vi "Nudge__LCR.vi"(7 "Nudging?":bool, 8 "error in (no error)":errorcluster, 9 "Nudge?":bool, 10 "NudgeValue":i32=1, 11 "Pict In":refnum<vi>) -> (0 "error out":errorcluster, 3 "PictOut":refnum<vi>)   [LabVIEW 2011, in "BooleanXControl__LCR.xctl"]
doc: "This VI will move the picture when needed to suggest a nudge."
uses:
  BooleanXControl__LCR.xctl
  <vilib>/Utility/miscctls.llb/LVPointTypeDef.ctl
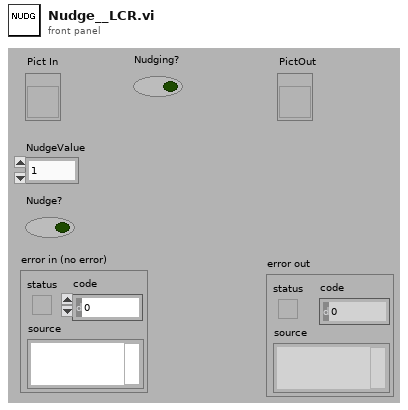
[diagram p1: front panel]
types:
  T1 = typedef "LVPointTypeDef.ctl" = cluster{"Horizontal":i16, "Vertical":i16}
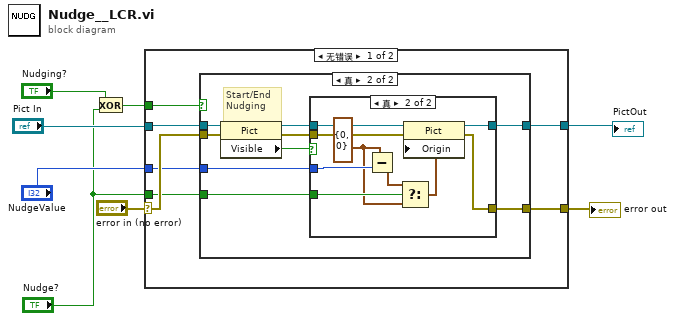
[diagram p0: block diagram]
diagram:
  n1 = Exclusive Or(1:"Nudge?", 2:"Nudging?") -> (0:w1:bool)
  n2 = case shown="无错误" "error in (no error)" {
    selector: "error in (no error)" -> [w14 w39]
    tunnel: [w12 w39] -> w7
    tunnel: "Pict In" -> [w15 w38]
    tunnel: "NudgeValue" -> [w13 _]
    tunnel: "Nudge?" -> [w11 _]
    tunnel: [w10 w38] -> w4
    tunnel: w1 -> [w9 _]
    frame No Error {
      n3 = case shown="真" w9 {
        tunnel: w15 -> [w17 w26]
        tunnel: w14 -> [w16 w25]
        tunnel: w13 -> [_ w21]
        tunnel: [w16 w20] -> w12
        tunnel: w11 -> [_ w19]
        tunnel: [w17 w18] -> w10
        frame False {
          # "Nudging status didn't change"
        }
        frame True {
          # "Start/End\nNudging"
          n4 = property class="Pict"(reference=w26, error in=w25) -> (reference out=w23:refnum<vi>, error out=w22:errorcluster, "Visible"=w24:bool)
          n5 = case shown="真" w24 {
            tunnel: w23 -> [w27 w35]
            tunnel: w22 -> [w28 w34]
            tunnel: w21 -> [_ w37]
            tunnel: [w28 w36] -> w20
            tunnel: w19 -> [_ w33]
            tunnel: [w27 w29] -> w18
            frame False {
            }
            frame True {
              w30 = T1 {"Horizontal"=0, "Vertical"=0} ("Origin")
              n6 = Subtract(x=w30, y=w37) -> (x-y=w32:cluster{"Horizontal":i32, "Vertical":i32})
              n7 = Select(t=w32, s=w33, f=w30) -> (s? t:f=w31:cluster{"Horizontal":i32, "Vertical":i32})
              n8 = property class="Pict"(reference=w35, error in=w34, "Origin"=w31) -> (reference out=w29:refnum<vi>, error out=w36:errorcluster)
            }
          }
        }
      }
    }
    frame Error {
    }
  }
  "error out" <- w7
  "PictOut" <- w4
